vi "Initialization VI.vi"(8 "error in (no error)":errorcluster, 10 "Custom XML":string, 11 "Device Item Ref in":T1 format="%.0x") -> (0 "error out":errorcluster, 3 "Device Item Ref out":T1 format="%.0x")   [LabVIEW 2016, in "LIN Frame Protection Addon System Explorer.lvlib"]
uses:
  LIN Frame Protection Addon System Explorer.lvlib
  <vilib>/NI Veristand/Custom Device API/Custom Device Item Ref.ctl
  Shared/SubVIs/GUID Lookup.vi
  <vilib>/NI Veristand/Custom Device API/Custom Device API.lvlib
  Shared/LIN Frame Protection Addon Shared.lvlib
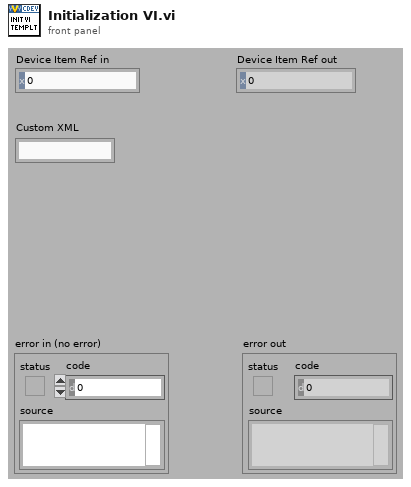
[diagram p1: front panel]
types:
  T1 = typedef "Custom Device API.lvlib/Custom Device Item Ref.ctl" = u64
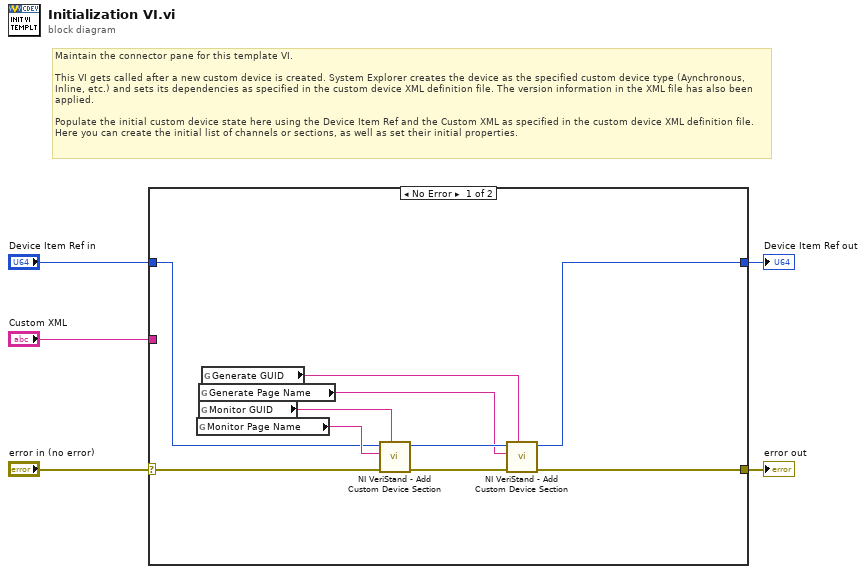
[diagram p0: block diagram]
diagram:
  # "Maintain the connector pane for this template VI.\n\nThis VI gets called after a new custom device is created. System Explorer creates the device as the specified custom device type (Aynchronous, Inline, etc.) and sets its dependencies as specified in the custom device XML definition file. The version information in the XML file has also been applied.\n\nPopulate the initial custom device state here using the Device Item Ref and the Custom XML as specified in the custom device XML definition file. Here you can create the initial list of channels or sections, as well as set their initial properties."
  n1 = case shown="No Error" "error in (no error)" {
    selector: "error in (no error)" -> [w15 w17]
    tunnel: [w12 w17] -> w5
    tunnel: [w6 w16] -> w3
    tunnel: "Device Item Ref in" -> [w7 w16]
    tunnel: "Custom XML" -> [_ _]
    frame No Error {
      n2 = global read "GUID Lookup.vi" "Monitor Page Name"() -> (w8:string)
      n3 = global read "GUID Lookup.vi" "Generate Page Name"() -> (w9:string)
      n4 = global read "GUID Lookup.vi" "Monitor GUID"() -> (w14:string)
      n5 = global read "GUID Lookup.vi" "Generate GUID"() -> (w10:string)
      n6 = call <vilib>:"NI VeriStand - Add Custom Device Section.vi"("GUID (Default Section)"=w14, "error in (no error)"=w15, "Section Name"=w8, "Parent Ref in"=w7) -> ("error out"=w13:errorcluster, "Parent Ref out"=w11:T1)  [unwired: 4 in, 2 out]
      n7 = call <vilib>:"NI VeriStand - Add Custom Device Section.vi"("GUID (Default Section)"=w10, "error in (no error)"=w13, "Section Name"=w9, "Parent Ref in"=w11) -> ("error out"=w12:errorcluster, "Parent Ref out"=w6:T1)  [unwired: 4 in, 2 out]
    }
    frame Error {
    }
  }
  "error out" <- w5
  "Device Item Ref out" <- w3
